vi "FilePowerSave.vi"(8 "error in (no error)":errorcluster, 10 "File Power":path, 11 "Data":refnum<vi>) -> (0 "error out":errorcluster)   [LabVIEW 2016]
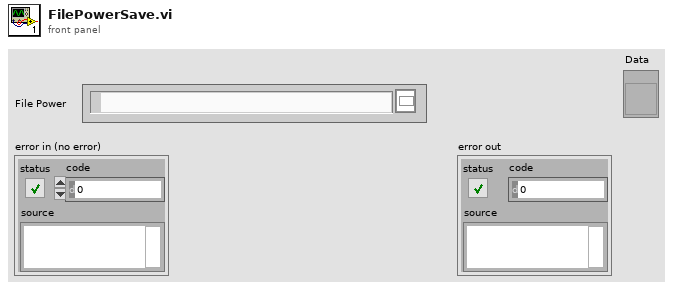
[diagram p1: front panel]
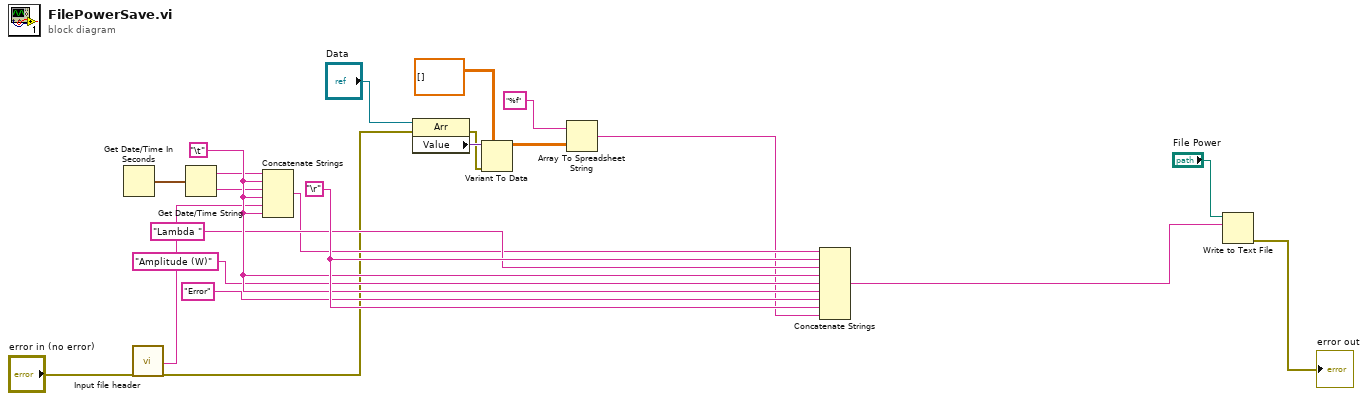
[diagram p0: block diagram]
diagram:
  w19 = "\r"
  w17 = "\t"
  n1 = Get Date/Time In Seconds() -> (seconds since 1Jan1904=w9:timestamp)
  n2 = call "Input file header"("error in (no error)"="error in (no error)") -> ("Header"=w12:string, "error out"=w5:errorcluster)  [unwired: 1 in, 16 out]
  n3 = Get Date/Time String(seconds (now)=w9) -> (date string=w10:string, time string=w11:string)  [unwired: 2 out]
  n4 = Concatenate Strings(w10, w17, w11, w17, w12, w17) -> (w14:string)
  n5 = property class="Arr"(reference="Data", error in=w5) -> (error out=w2:errorcluster, "Value"=w4:variant)  [unwired: 1 out]
  n6 = Variant To Data(error in=w2, type=dbl[][] [], Variant=w4) -> (data=w1:dbl[][])  [unwired: 1 out]
  n7 = Array To Spreadsheet String(array=w1, 3:"%f") -> (spreadsheet string=w7:string)  [unwired: 1 in]
  n8 = Concatenate Strings(w14, w19, "Lambda ", w17, "Amplitude (W)", w17, "Error", w19, w7) -> (w20:string)
  n9 = Write to Text File(file (use dialog)="File Power", text=w20) -> (error out=→"error out":errorcluster)  [unwired: 2 in, 2 out]
